vi "Actor Core.vi"(8 "error in":errorcluster, 11 "Nested in":refnum<class "Database Provider.lvclass">) -> (0 "error out":errorcluster, 3 "Actor out":refnum<class "Actor.lvclass">)   [LabVIEW 2024, in "Database Provider.lvlib" / "Database Provider.lvclass"]
doc: "(<B>Filename</B>: Actor Framework.lvlib:Actor.lvclass:Actor Core.vi)\n\nReceives messages to the actor, reacts to them, and initiates any error handling that may shut the actor down.\n\nDescendant classes may override this VI to append parallel tasks for the actor to complete while it handles messages. Overrides use the Call Parent Method node."
uses:
  Database Provider.lvclass
  <vilib>/ActorFramework/Actor/Actor.lvclass
  Database Provider.lvclass/Database Provider.ctl
  <vilib>/Utility/miscctls.llb/LVRowAndColumnUnsignedTypeDef.ctl
  <vilib>/ActorFramework/Actor/Actor.lvclass/Actor.ctl
  Database Provider Messages/Read Database Msg/Read Database Msg.lvclass/Read Database Msg.ctl
  <vilib>/ActorFramework/Message Enqueuer/Message Enqueuer.lvclass/Message Enqueuer.ctl
  Database Provider Messages/Read Instr CFGs Msg/Read Instr CFGs Msg.lvclass/Read Instr CFGs Msg.ctl
  IConfiguration UI Actor/IConfiguration UI Actor Messages/Add Instr CFG Msg/Add Instr CFG Msg.lvclass/Add Instr CFG Msg.ctl
  IConfiguration UI Actor/IConfiguration UI Actor Messages/Set Virt Instr CFG Msg/Set Virt Instr CFG Msg.lvclass/Set Virt Instr CFG Msg.ctl
  IConfiguration UI Actor/IConfiguration UI Actor Messages/Set Series CFG Msg/Set Series CFG Msg.lvclass/Set Series CFG Msg.ctl
  <vilib>/ActorFramework/Message Enqueuer/Enqueue.vi
  Database Provider Messages/Read Database Msg/Read Database Msg.lvclass
  Database Provider Messages/Read Instr CFGs Msg/Read Instr CFGs Msg.lvclass
  IConfiguration UI Actor/IConfiguration UI Actor Messages/Add Instr CFG Msg/Add Instr CFG Msg.lvclass
  IConfiguration UI Actor/IConfiguration UI Actor Messages/Set Virt Instr CFG Msg/Set Virt Instr CFG Msg.lvclass
  IConfiguration UI Actor/IConfiguration UI Actor Messages/Set Series CFG Msg/Set Series CFG Msg.lvclass
  <vilib>/Utility/LVClass/Get LV Class Name.vi
  <resource>/AFDebug/Generate Trace for Message.vi
  <vilib>/ActorFramework/Message Priority Queue/Priority Enqueue.vi
  <vilib>/MGI/Panel Manager/Panel Actor/Panel Actor/Panel Actor.lvclass
panel:
  in  "Load":bool
  in  "Series CFGs":string[][](table)
  in  "Series Instr CFGs":string[][](table)
  in  "DB File Path":path=path "D:/git/HAL/Configurator/CFG Provider/Database/configs.db"
  in  "Open Button":bool
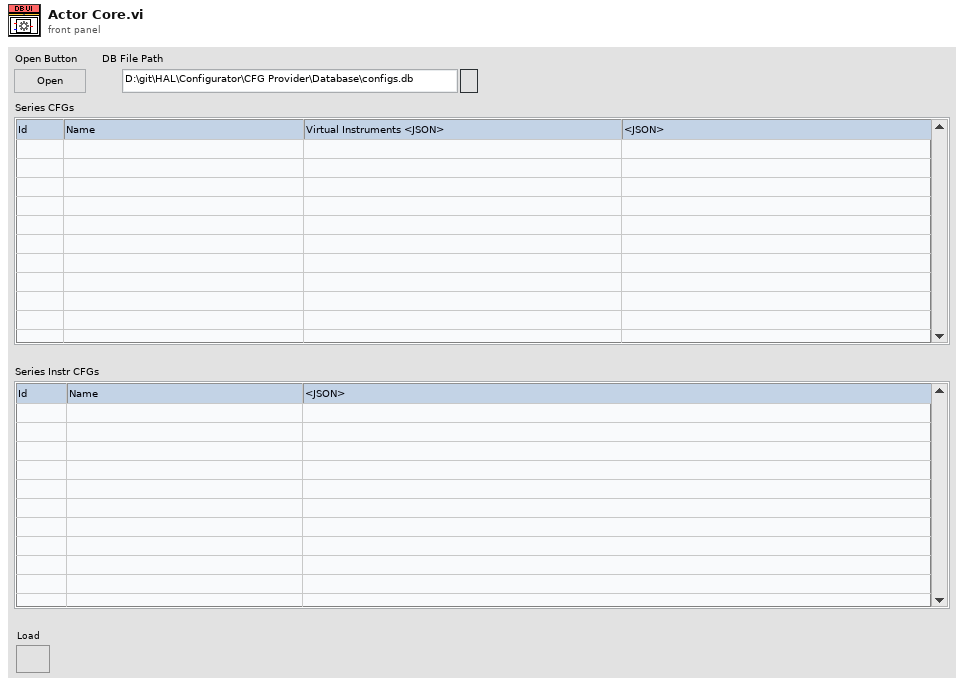
[diagram p1: front panel]
types:
  T1 = cluster{"Series":string, "Virt Instrs":string, "Instrs":string[]}
  T2 = typedef "LVRowAndColumnUnsignedTypeDef.ctl" = cluster{"Row":u32, "Column":u32}
  T3 = cluster{"Pnl Actor":refnum<event-registration>, "Event Registration Refnum":refnum<event-registration>}
  T4 = typedef "LVPoint32TypeDef.ctl" = cluster{"Horizontal":i32, "Vertical":i32}
  T5 = typedef "LVRowAndColumnTypeDef.ctl" = cluster{"Row":i32, "Column":i32}
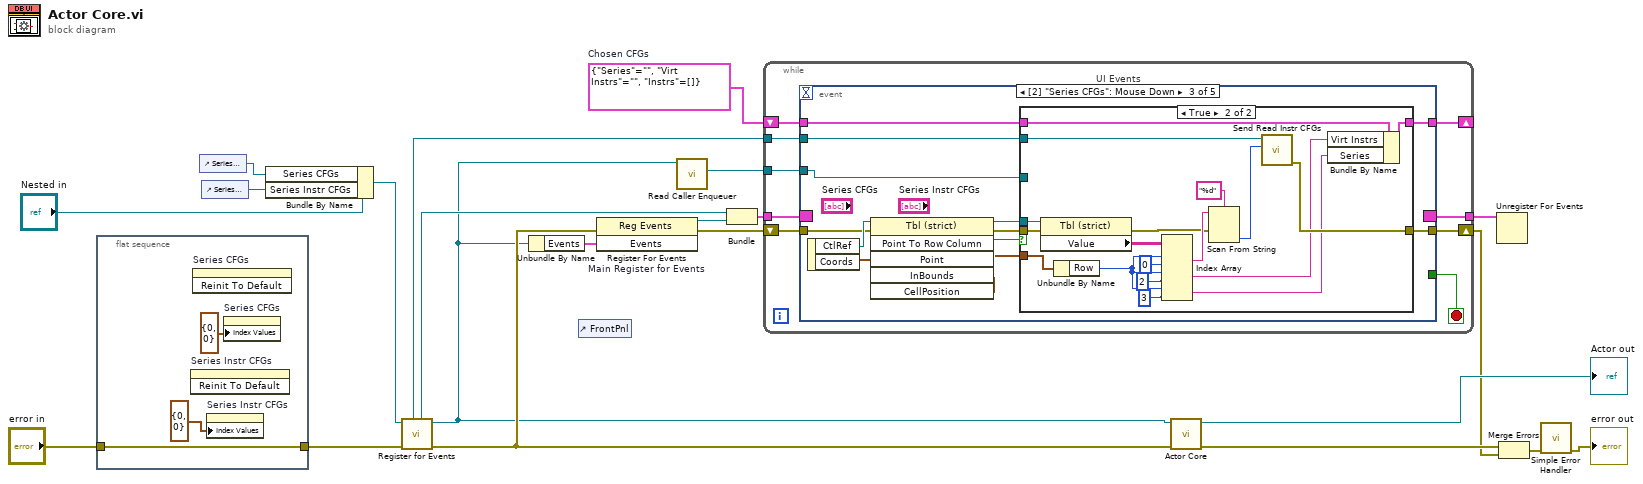
[diagram p0: block diagram]
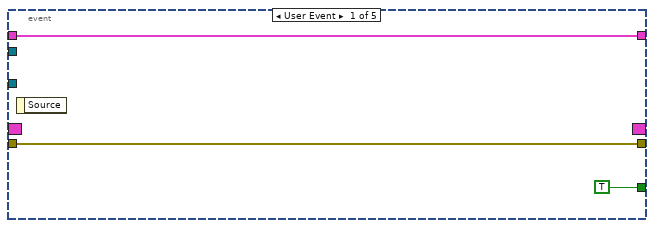
[diagram p2: hidden frame]
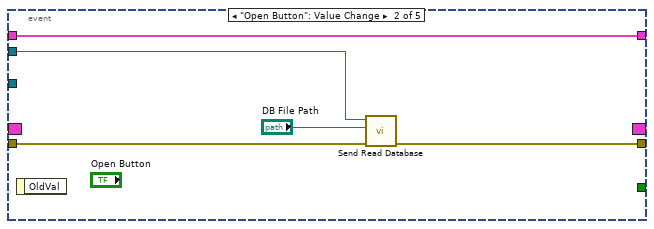
[diagram p3: hidden frame]
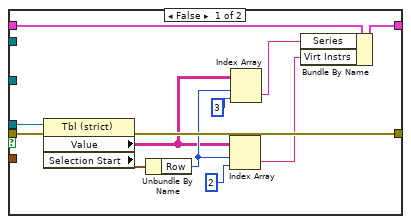
[diagram p4: hidden frame]
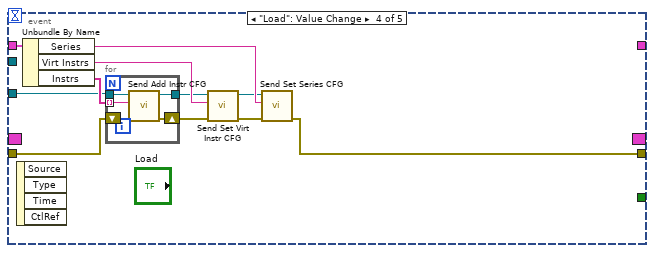
[diagram p5: hidden frame]
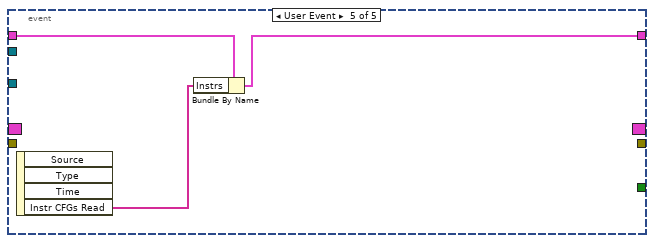
[diagram p6: hidden frame]
diagram:
  w13 = T1 {"Series"="", "Virt Instrs"="", "Instrs"=[]}  # Chosen CFGs
  n1 = flat-sequence {
    tunnel: "error in" -> [w25]
    tunnel: [w25] -> w1
    frame #0 {
      n2 = invoke on="Series Instr CFGs" class="Tbl (strict)" method="Reinit To Default"() -> ()  [unwired: 3 in, 3 out]
      n3 = invoke on="Series CFGs" class="Tbl (strict)" method="Reinit To Default"() -> ()  [unwired: 3 in, 3 out]
      n4 = property on="Series Instr CFGs" class="Tbl (strict)"("Index Values"=T2 {"Row"=0, "Column"=0}) -> ()  [unwired: 2 in, 2 out]
      n5 = property on="Series CFGs" class="Tbl (strict)"("Index Values"=T2 {"Row"=0, "Column"=0}) -> ()  [unwired: 2 in, 2 out]
    }
  }
  n6 = control-ref of="Series CFGs"() -> (w10:refnum<vi>)
  n7 = control-ref of="Series Instr CFGs"() -> (w15:refnum<vi>)
  n8 = Bundle By Name(cluster="Nested in", "Series CFGs"=w10, "Series Instr CFGs"=w15) -> (w3:refnum<class "Database Provider.lvclass">)
  n9 = call <vilib>:"Register for Events.vi"("Error In"=w1, "Panel Actor in"=w3) -> ("Error Out"=w11:errorcluster, "Panel Actor out"=w5:refnum<class "Database Provider.lvclass">, "Pnl Actor"=w16:refnum<event-registration>, "Self Enqueuer"=w18:refnum<class "Message Enqueuer.lvclass">)  [unwired: 6 in]
  n10 = Unbundle By Name(w5) -> ("Events"=w19:cluster{"Instr CFGs Read":refnum<user-event>})
  n11 = control-ref of="FrontPnl"() -> ()  [unwired: 1 out]
  n12 = register-events "Main Register for Events"(error in=w11, w19) -> (reference out=w20:refnum<event-registration>, error out=w12:errorcluster)  [unwired: 1 in]
  n13 = call <vilib>:"Read Caller Enqueuer.vi"("Actor"=w5) -> ("Caller Enqueuer"=w14:refnum<class "Message Enqueuer.lvclass">)  [unwired: 10 in]
  n14 = Bundle("Pnl Actor"=w16, "Event Registration Refnum"=w20) -> (w17:T3)  [unwired: 1 in]
  n15 = while {
    tunnel: w17 -> [w34]
    tunnel: w18 -> [w32]
    tunnel: w14 -> [w31]
    shift-right: [w29] -> _
    shift-left: w13 -> [w30]
    shift-right: [w27] -> w8
    shift-left: w12 -> [w28]
    tunnel: [w26] -> w6
    stop <- w33 stop-if-true
    n16 = event "UI Events" shown="[2] \"Series CFGs\": Mouse Down" {
      selector: w34 -> [_ _ _ _ _]
      dyn-events: [_ _ _ _ _] -> w26
      timeout: _ -> [_ _ _ _ _]
      tunnel: [TRUE _ _ _ _] -> w33
      tunnel: w32 -> [_ w42 w52 _ _]
      tunnel: w31 -> [_ _ w43 w92 _]
      tunnel: w30 -> [w36 w38 w49 w95 w103]
      tunnel: [w36 w38 w48 _ w101] -> w29
      tunnel: w28 -> [w35 w40 w46 w86 _]
      tunnel: [w35 w39 w44 w85 _] -> w27
      event User Event {
        n17 = event-data() -> ()  [unwired: 1 in, 1 out]
      }
      event "Open Button": Value Change {
        n18 = event-data() -> ()  [unwired: 1 in, 1 out]
        n19 = call "Send Read Database.vi"("error in (no error)"=w40, "DB File Path"="DB File Path", "Message Enqueuer"=w42) -> ("error out"=w39:errorcluster)  [unwired: 7 in, 1 out]
      }
      event "Series CFGs": Mouse Down {
        n20 = event-data() -> ("CtlRef"=w51:refnum<vi>, "Coords"=w50:T4)  [unwired: 1 in]
        n21 = invoke class="Tbl (strict)" method="Point To Row Column"(reference=w51, error in=w46, "Point"=w50) -> (reference out=w47:refnum<vi>, error out=w45:errorcluster, "InBounds"=w54:bool, "CellPosition"=w53:T5)  [unwired: 3 in, 2 out]
        n22 = case shown="True" w54 {
          tunnel: w53 -> [_ w84]
          tunnel: w52 -> [_ w77]
          tunnel: w49 -> [w66 w82]
          tunnel: [w62 w81] -> w48
          tunnel: w47 -> [w65 w80]
          tunnel: w45 -> [w61 w79]
          tunnel: [w60 w73] -> w44
          tunnel: w43 -> [_ _]
          frame False {
            n23 = property class="Tbl (strict)"(reference=w65, error in=w61) -> (error out=w60:errorcluster, "Value"=w58:string[][], "Selection Start"=w64:T5)  [unwired: 1 out]
            n24 = Unbundle By Name(w64) -> ("Row"=w59:i32)
            n25 = Index Array(array=w58, index (row)=w59, index (col)=2) -> (element=w56:string)
            n26 = Index Array(array=w58, index (row)=w59, index (col)=3) -> (element=w55:string)
            n27 = Bundle By Name(cluster=w66, "Series"=w55, "Virt Instrs"=w56) -> (w62:T1)
          }
          frame True {
            n28 = property class="Tbl (strict)"(reference=w80, error in=w79) -> (error out=w71:errorcluster, "Value"=w78:string[][])  [unwired: 1 out]
            n29 = Unbundle By Name(w84) -> ("Row"=w76:i32)
            n30 = Index Array(array=w78, index (row) #1=w76, index (col) #1=0 ("index (col)"), index (row) #2=w76, index (col) #2=2 ("index (col)"), index (row) #3=w76, index (col) #3=3 ("index (col)")) -> (element #1=w72:string, element #2=w67:string, element #3=w68:string)
            n31 = Scan From String(format string="%d", input string=w72, error in=w71) -> (output 1=w70:u32)  [unwired: 2 in, 3 out]
            n32 = call "Send Read Instr CFGs.vi"("Series Id"=w70, "Message Enqueuer"=w77) -> ("error out"=w73:errorcluster)  [unwired: 8 in, 1 out]
            n33 = Bundle By Name(cluster=w82, "Virt Instrs"=w67, "Series"=w68) -> (w81:T1)
          }
        }
      }
      event "Load": Value Change {
        n34 = event-data() -> ()  [unwired: 1 in, 4 out]
        n35 = Unbundle By Name(w95) -> ("Series"=w90:string, "Virt Instrs"=w94:string, "Instrs"=w93:string[])
        n36 = for {
          tunnel: w93 -> [w100] mode=indexing
          tunnel: w92 -> [w99]
          tunnel: [w98] -> w91
          shift-right: [w97] -> w88
          shift-left: w86 -> [w96]
          n37 = call "Send Add Instr CFG.vi"("error in (no error)"=w96, "Instr Configuration"=w100, "Message Enqueuer"=w99) -> ("error out"=w97:errorcluster, "Message Enqueuer out"=w98:refnum<class "Message Enqueuer.lvclass">)  [unwired: 7 in]
        }
        n38 = call "Send Set Virt Instr CFG.vi"("error in (no error)"=w88, "Virt Instr CFG"=w94, "Message Enqueuer"=w91) -> ("error out"=w87:errorcluster, "Message Enqueuer out"=w89:refnum<class "Message Enqueuer.lvclass">)  [unwired: 7 in]
        n39 = call "Send Set Series CFG.vi"("error in (no error)"=w87, "Series CFG"=w90, "Message Enqueuer"=w89) -> ("error out"=w85:errorcluster)  [unwired: 7 in, 1 out]
      }
      event User Event {
        n40 = event-data() -> ("Instr CFGs Read"=w102:string[])  [unwired: 1 in, 3 out]
        n41 = Bundle By Name(cluster=w103, "Instrs"=w102) -> (w101:T1)
      }
    }
  }
  n42 = call-parent "Actor Core.vi"("error in"=w11, "Panel Actor in"=w5) -> ("error out"=w22:errorcluster, "Actor out"=→"Actor out":refnum<class "Actor.lvclass">)  [unwired: 8 in]
  n43 = Unregister For Events(event registration refnum=w6) -> ()  [unwired: 1 in, 1 out]
  n44 = Merge Errors(w22, w8) -> (w9:errorcluster)
  n45 = call <vilib>:"Simple Error Handler.vi"("error in (no error)"=w9) -> ("error out"=→"error out":errorcluster)  [unwired: 4 in, 4 out]
